vi "WithTestSuite_Empty.vi"() -> ()   [LabVIEW 2017, in "ResultTree.Tests.lvlib" / "Clear.lvlib"]
uses:
  Clear.lvlib
  ResultTree/ResultTree.lvclass
  Assertion/Assertion.lvlib
panel:
  out "error out":errorcluster
  in  "Tree":string(tree)
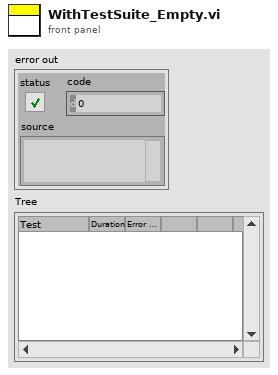
[diagram p1: front panel]
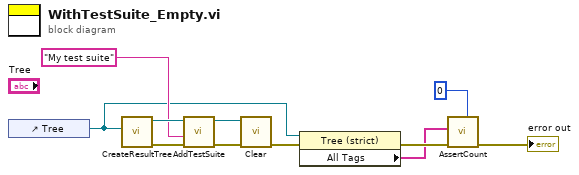
[diagram p0: block diagram]
diagram:
  n1 = control-ref of="Tree"() -> (w6:refnum<vi>)
  n2 = call "CreateResultTree.vi"("Tree Refnum"=w6) -> ("error out"=w11:errorcluster, "ResultTree out"=w9:refnum<class "ResultTree.lvclass">)  [unwired: 9 in]
  n3 = call "AddTestSuite.vi"("error in (no error)"=w11, "Name"="My test suite", "ResultTree in"=w9) -> ("error out"=w10:errorcluster, "ResultTree out"=w7:refnum<class "ResultTree.lvclass">)  [unwired: 6 in, 1 out]
  n4 = call "Clear.vi"("error in (no error)"=w10, "ResultTree in"=w7) -> ("error out"=w5:errorcluster)  [unwired: 8 in, 1 out]
  n5 = property class="Tree (strict)"(reference=w6, error in=w5) -> (error out=w4:errorcluster, "All Tags"=w2:string[])  [unwired: 1 out]
  n6 = call "AssertCount.vi"("Expected"=0, "error in (no error)"=w4, "Haystack"=w2) -> ("error out"=→"error out":errorcluster)  [unwired: 8 in]
